vi "EOL Breakin Set Switch Output.vi"(8 "Error In":errorcluster, 10 "Current Motion":T2, 11 "Switch Output Array":T1[](array[typedef])) -> (0 "Error Out":errorcluster)   [LabVIEW 2018]
uses:
  05.UserVI's/type defs/EOL Global Digital Output Control.ctl
  05.UserVI's/type defs/EOL Global Digital Output Cluster Control.ctl
  02.Type Def's/All Motions.ctl
  02.Type Def's/All Switch Configuration Cluster.ctl
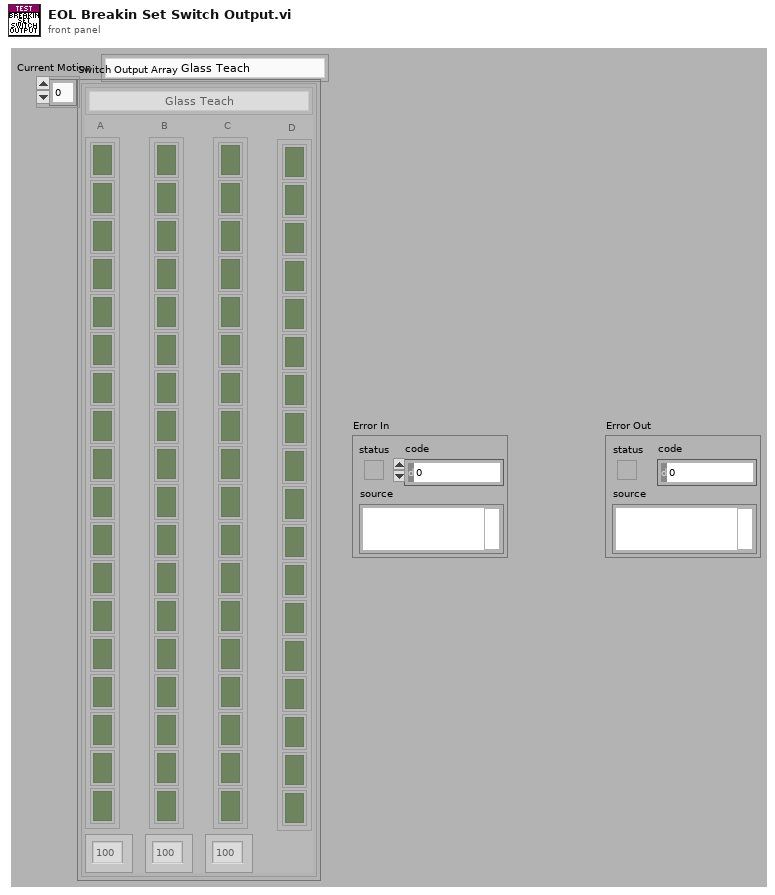
[diagram p1: front panel]
types:
  T1 = typedef "All Switch Configuration Cluster.ctl" = cluster{"All Motions":T2, "A":bool[], "B":bool[], "C":bool[], "D":bool[], "A activation time (ms)":u32, "B activation time (ms)":u32, "C activation time (ms)":u32}
  T2 = typedef "All Motions.ctl" = enum16{"Glass Teach", "Glass Slide Open", "Glass Slide Close", "Glass Vent Open", "Glass Vent Close", "Sunshade Teach", "Sunshade Open", "Sunshade Close", "Idle", "Sunshade Open 2", "Sunshade Close 2", "Glass Slide Open Sunshade Open", "Glass Slide Open Sunshade Close", "Glass Slide Close Sunshade Open", "Glass Slide Close Sunshade Close", "Glass Vent Open Sunshade Open", "Glass Vent Open Sunshade Close", "Glass Vent Close Sunshade Open", "Glass Vent Close Sunshade Close", "Express Glass Slide Open", "Express Glass Slide Close", "Express Glass Vent Open", "Express Glass Vent Close", "Express Sunshade Open", "Express Sunshade Close", "Express Sunshade Open 2", "Express Sunshade Close 2", "Express Glass Slide Open Sunshade Open", "Express Glass Slide Open Sunshade Close", "Express Glass Slide Close Sunshade Open", "Express Glass Slide Close Sunshade Close", "Express Glass Vent Open Sunshade Open", "Express Glass Vent Open Sunshade Close", "Express Glass Vent Close Sunshade Open", "Express Glass Vent Close Sunshade Close", "Goto Position Glass", "Goto Position Sunshade", "Sunshade Teach 2"}
  T3 = typedef "EOL Global Digital Output Control.ctl" = enum16{"Prerun Battery", "Prerun Ignition High", "Prerun Switch 1", "Prerun Switch 2", "Prerun Switch 3", "Prerun Select NI LIN", "Prerun Switch 4", "Prerun Switch 5", "Prerun Switch 6", "Prerun Ignition Low", "Prerun Glass Analog Switch 1", "Prerun Glass Analog Switch 2", "Prerun Glass Analog Switch 3", "Prerun Glass Analog Switch 4", "Prerun Sunshade Analog Switch 1", "Prerun Sunshade Analog Switch 2", "Prerun Sunshade Analog Switch 3", "Prerun Sunshade Analog Switch 4", "Prerun Select RS232 LIN", "Prerun Select RS232", "Prerun Select CAN", "Prerun Park/Enable", "Prerun Communications Power", "Prerun BMW Glass Motor Relay 1", "Prerun BMW Glass Motor Relay 2", "Prerun BMW Sunshade Motor Relay 1", "Prerun BMW Sunshade Motor Relay 2", "Prerun Spare 1", "Prerun Spare 2", "Prerun Spare 3", "Prerun Spare 4", "Prerun Spare 5", "Audit Battery", "Audit Ignition High", "Audit Ignition Low", "Audit Switch 1", "Audit Switch 2", "Audit Switch 3", "Audit Switch 4", "Audit Switch 5", "Audit Switch 6", "Audit Glass Analog Switch 1", "Audit Glass Analog Switch 2", "Audit Glass Analog Switch 3", "Audit Glass Analog Switch 4", "Audit Sunshade Analog Switch 1", "Audit Sunshade Analog Switch 2", "Audit Sunshade Analog Switch 3", "Audit Sunshade Analog Switch 4", "Audit Select NI LIN", "Audit Select RS232 LIN", "Audit Select RS232", "Audit Select CAN", "Audit Park/Enable", "Audit Communications Power", "Audit BMW Glass Motor Relay 1", "Audit BMW Glass Motor Relay 2", "Audit BMW Sunshade Motor Relay 1", "Audit BMW Sunshade Motor Relay 2", "Audit Spare 1", "Audit Spare 2", "Audit Spare 3", "Audit Spare 4", "Audit Spare 5", "Repair Battery", "Repair Ignition High", "Repair Switch 1", "Repair Switch 2", "Repair Select NI LIN", "Repair Ignition Low", "Repair Switch 3", "Repair Switch 4", "Repair Switch 5", "Repair Switch 6", "Repair Glass Analog Switch 1", "Repair Glass Analog Switch 2", "Repair Glass Analog Switch 3", "Repair Glass Analog Switch 4", "Repair Sunshade Analog Switch 1", "Repair Sunshade Analog Switch 2", "Repair Sunshade Analog Switch 3", "Repair Sunshade Analog Switch 4", "Repair Select RS232 LIN", "Repair Select RS232", "Repair Select CAN", "Repair Select Park/Enable", "Repair Communications Power", "Repair BMW Glass Motor Relay 1", "Repair BMW Glass Motor Relay 2", "Repair BMW Sunshade Motor Relay 1", "Repair BMW Sunshade Motor Relay 2", "Repair Spare 1", "Repair Spare 2", "Repair Spare 3", "Repair Spare 4", "Repair Spare 5", "Breakin Battery", "Breakin Igntiion High", "Breakin Ignition Low", "Breakin Switch 1", "Breakin Switch 2", "Breakin Switch 3", "Breakin Switch 4", "Breakin Switch 5", "Breakin Switch 6", "Breakin Glass Analog Switch 1", "Breakin Glass Analog Switch 2", "Breakin Glass Analog Switch 3", "Breakin Glass Analog Switch 4", "Breakin Sunshade Analog Switch 1", "Breakin Sunshade Analog Switch 2", "Breakin Sunshade Analog Switch 3", "Breakin Sunshade Analog Switch 4", "Breakin Select NI LIN", "Breakin Select RS232 LIN", "Breakin Select RS232", "Breakin Select CAN", "Breakin Park/Enable", "Breakin Communications Power", "Breakin BMW Glass Motor Relay 1", "Breakin BMW Glass Motor Relay 2", "Breakin BMW Sunshade Motor Relay 1", "Breakin BMW Sunshade Motor Relay 2", "Breakin Spare 1", "Breakin Spare 2", "Breakin Spare 3", "Breakin Spare 4", "Breakin Spare 5", "Not Implemented"}
  T4 = typedef "EOL Global Digital Output Cluster Control.ctl" = cluster{"Status":bool, "Global DO Ch":T3}
  T5 = enum16{"Init", "Write", "Write All", "Clear All", "Stop"}
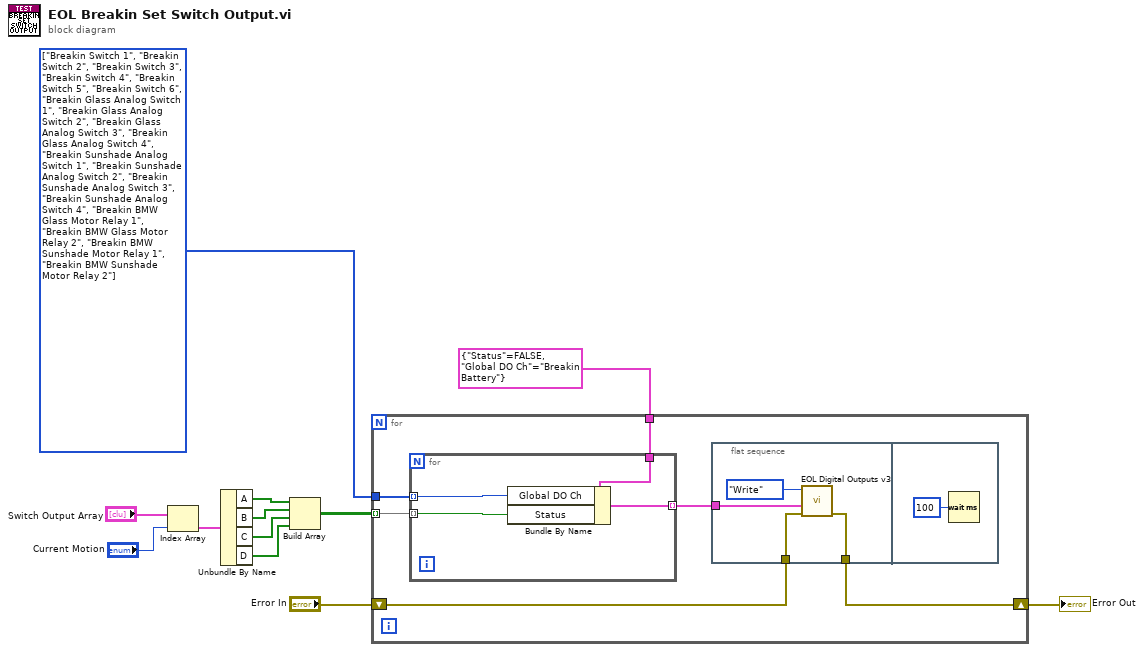
[diagram p0: block diagram]
diagram:
  w4 = T3[] [enum."Breakin Switch 1", enum."Breakin Switch 2", enum."Breakin Switch 3", enum."Breakin Switch 4", enum."Breakin Switch 5", enum."Breakin Switch 6", enum."Breakin Glass Analog Switch 1", enum."Breakin Glass Analog Switch 2", enum."Breakin Glass Analog Switch 3", enum."Breakin Glass Analog Switch 4", enum."Breakin Sunshade Analog Switch 1", enum."Breakin Sunshade Analog Switch 2", enum."Breakin Sunshade Analog Switch 3", enum."Breakin Sunshade Analog Switch 4", enum."Breakin BMW Glass Motor Relay 1", enum."Breakin BMW Glass Motor Relay 2", enum."Breakin BMW Sunshade Motor Relay 1", enum."Breakin BMW Sunshade Motor Relay 2"] items=["Prerun Battery", "Prerun Ignition High", "Prerun Switch 1", "Prerun Switch 2", "Prerun Switch 3", "Prerun Select NI LIN", "Prerun Switch 4", "Prerun Switch 5", "Prerun Switch 6", "Prerun Ignition Low", "Prerun Glass Analog Switch 1", "Prerun Glass Analog Switch 2", "Prerun Glass Analog Switch 3", "Prerun Glass Analog Switch 4", "Prerun Sunshade Analog Switch 1", "Prerun Sunshade Analog Switch 2", "Prerun Sunshade Analog Switch 3", "Prerun Sunshade Analog Switch 4", "Prerun Select RS232 LIN", "Prerun Select RS232", "Prerun Select CAN", "Prerun Park/Enable", "Prerun Communications Power", "Prerun BMW Glass Motor Relay 1", "Prerun BMW Glass Motor Relay 2", "Prerun BMW Sunshade Motor Relay 1", "Prerun BMW Sunshade Motor Relay 2", "Prerun Spare 1", "Prerun Spare 2", "Prerun Spare 3", "Prerun Spare 4", "Prerun Spare 5", "Audit Battery", "Audit Ignition High", "Audit Ignition Low", "Audit Switch 1", "Audit Switch 2", "Audit Switch 3", "Audit Switch 4", "Audit Switch 5", "Audit Switch 6", "Audit Glass Analog Switch 1", "Audit Glass Analog Switch 2", "Audit Glass Analog Switch 3", "Audit Glass Analog Switch 4", "Audit Sunshade Analog Switch 1", "Audit Sunshade Analog Switch 2", "Audit Sunshade Analog Switch 3", "Audit Sunshade Analog Switch 4", "Audit Select NI LIN", "Audit Select RS232 LIN", "Audit Select RS232", "Audit Select CAN", "Audit Park/Enable", "Audit Communications Power", "Audit BMW Glass Motor Relay 1", "Audit BMW Glass Motor Relay 2", "Audit BMW Sunshade Motor Relay 1", "Audit BMW Sunshade Motor Relay 2", "Audit Spare 1", "Audit Spare 2", "Audit Spare 3", "Audit Spare 4", "Audit Spare 5", "Repair Battery", "Repair Ignition High", "Repair Switch 1", "Repair Switch 2", "Repair Select NI LIN", "Repair Ignition Low", "Repair Switch 3", "Repair Switch 4", "Repair Switch 5", "Repair Switch 6", "Repair Glass Analog Switch 1", "Repair Glass Analog Switch 2", "Repair Glass Analog Switch 3", "Repair Glass Analog Switch 4", "Repair Sunshade Analog Switch 1", "Repair Sunshade Analog Switch 2", "Repair Sunshade Analog Switch 3", "Repair Sunshade Analog Switch 4", "Repair Select RS232 LIN", "Repair Select RS232", "Repair Select CAN", "Repair Select Park/Enable", "Repair Communications Power", "Repair BMW Glass Motor Relay 1", "Repair BMW Glass Motor Relay 2", "Repair BMW Sunshade Motor Relay 1", "Repair BMW Sunshade Motor Relay 2", "Repair Spare 1", "Repair Spare 2", "Repair Spare 3", "Repair Spare 4", "Repair Spare 5", "Breakin Battery", "Breakin Igntiion High", "Breakin Ignition Low", "Breakin Switch 1", "Breakin Switch 2", "Breakin Switch 3", "Breakin Switch 4", "Breakin Switch 5", "Breakin Switch 6", "Breakin Glass Analog Switch 1", "Breakin Glass Analog Switch 2", "Breakin Glass Analog Switch 3", "Breakin Glass Analog Switch 4", "Breakin Sunshade Analog Switch 1", "Breakin Sunshade Analog Switch 2", "Breakin Sunshade Analog Switch 3", "Breakin Sunshade Analog Switch 4", "Breakin Select NI LIN", "Breakin Select RS232 LIN", "Breakin Select RS232", "Breakin Select CAN", "Breakin Park/Enable", "Breakin Communications Power", "Breakin BMW Glass Motor Relay 1", "Breakin BMW Glass Motor Relay 2", "Breakin BMW Sunshade Motor Relay 1", "Breakin BMW Sunshade Motor Relay 2", "Breakin Spare 1", "Breakin Spare 2", "Breakin Spare 3", "Breakin Spare 4", "Breakin Spare 5", "Not Implemented"]
  n1 = Index Array(array="Switch Output Array", index="Current Motion") -> (element=w10:T1)
  n2 = Unbundle By Name(w10) -> ("A"=w9:bool[], "B"=w8:bool[], "C"=w7:bool[], "D"=w6:bool[])
  n3 = Build Array(w9, w8, w7, w6) -> (w5:bool[][])
  n4 = for {
    tunnel: w5 -> [w18] mode=indexing
    tunnel: w4 -> [w17]
    tunnel: T4 {"Status"=FALSE, "Global DO Ch"=enum."Breakin Battery"} ("Cluster") -> [w16]
    shift-right: [w13] -> w1
    shift-left: "Error In" -> [w14]
    n5 = for {
      tunnel: w18 -> [w25] mode=indexing
      tunnel: w17 -> [w26] mode=indexing
      tunnel: w16 -> [w27]
      tunnel: [w24] -> w15 mode=indexing
      n6 = Bundle By Name(cluster=w27, "Global DO Ch"=w26, "Status"=w25) -> (w24:T4)
    }
    n7 = flat-sequence {
      tunnel: w15 -> [w21]
      tunnel: w14 -> [w20]
      tunnel: [w19] -> w13
      frame #0 {
        n8 = call "EOL Digital Outputs v3.vi"("Error In"=w20, "DO Status"=w21, "Mode"=T5."Write") -> ("Error Out"=w19:errorcluster)  [unwired: 7 in, 1 out]
      }
      frame #1 {
        n9 = Wait (ms)(milliseconds to wait=u32 100) -> ()  [unwired: 1 out]
      }
    }
  }
  "Error Out" <- w1
